vi "DateTimeInteger_to_TimeStamp.vi"(0 "Month":i32, 1 "Day of Month":i32, 2 "Year":i32, 3 "Hour":i32, 4 "Minute":i32, 5 "Second":i32) -> (17 "Time Stamp":timestamp)   [LabVIEW 2012]
panel:
  in  "date time rec":T1
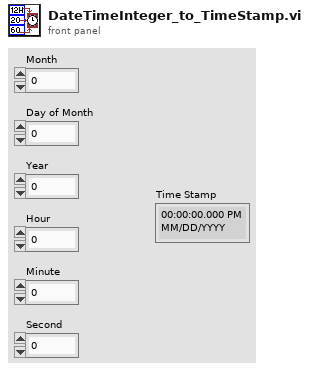
[diagram p1: front panel]
types:
  T1 = cluster{"second":i32, "minute":i32, "hour":i32, "day of month":i32, "month":i32, "year":i32, "day of week":i32, "day of year":i32, "is DST":i32}
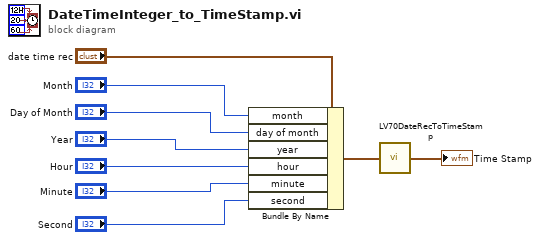
[diagram p0: block diagram]
diagram:
  n1 = Bundle By Name(cluster="date time rec", "month"="Month", "day of month"="Day of Month", "year"="Year", "hour"="Hour", "minute"="Minute", "second"="Second") -> (w7:T1)
  n2 = call <vilib>:"LV70DateRecToTimeStamp.vi"("date time rec"=w7) -> ("Time Stamp"=→"Time Stamp":timestamp)
